vi "Get Process UEs.vi"(11 "Process in":refnum<class "Process.lvclass">) -> (2 "Process UEs":refnum<user-event>[](array[refnum]), 3 "Process out":refnum<class "Process.lvclass">)   [LabVIEW 2019, in "TimingDRV Engine.lvlib" / "Process.lvclass"]
uses:
  Process.lvclass
  TypeDefs/Update.ctl
  Process.lvclass/Process.ctl
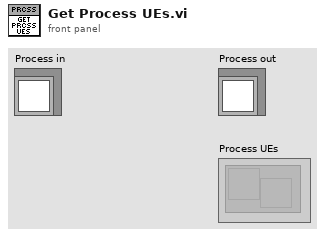
[diagram p1: front panel]
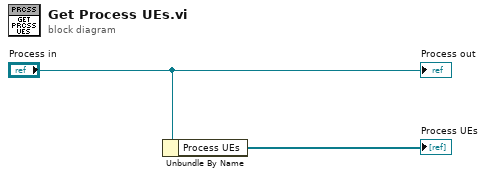
[diagram p0: block diagram]
diagram:
  n1 = Unbundle By Name("Process in") -> ("Process UEs"=→"Process UEs":refnum<user-event>[])
  "Process out" <- "Process in"
